vi "Get Joystick Values.vi"(8 "error in (no error)":errorcluster, 11 "One Driver in":refnum<class "One Driver.lvclass">) -> (0 "error out":errorcluster, 2 "Joystick Data":T1, 3 "One Driver out":refnum<class "One Driver.lvclass">)   [LabVIEW 2018, in "Joysticks.lvlib" / "One Driver.lvclass"]
doc: "Use this method to get the joystick values in a cluster you can use for your application.\n\nModify the Type Def that this VI resturns to fit the controls needed for the robot."
uses:
  One Driver.lvclass
  C:/Users/Public/Documents/2019DeepSpace/Classes/Joysticks/Joysticks.lvclass
  Controls/JoystickData.ctl
  One Driver.lvclass/One Driver.ctl
  Joysticks.lvclass/Joysticks.ctl
  Public Methods/Read Sensitivity(x).vi
  Public Methods/Read Sensitivity(y).vi
  <vilib>/Rock Robotics/WPI/Utilities/WPI_GetSetVariantRefNum.vi
  Private Methods/POV Conditioning.vi
  Joysticks.lvclass
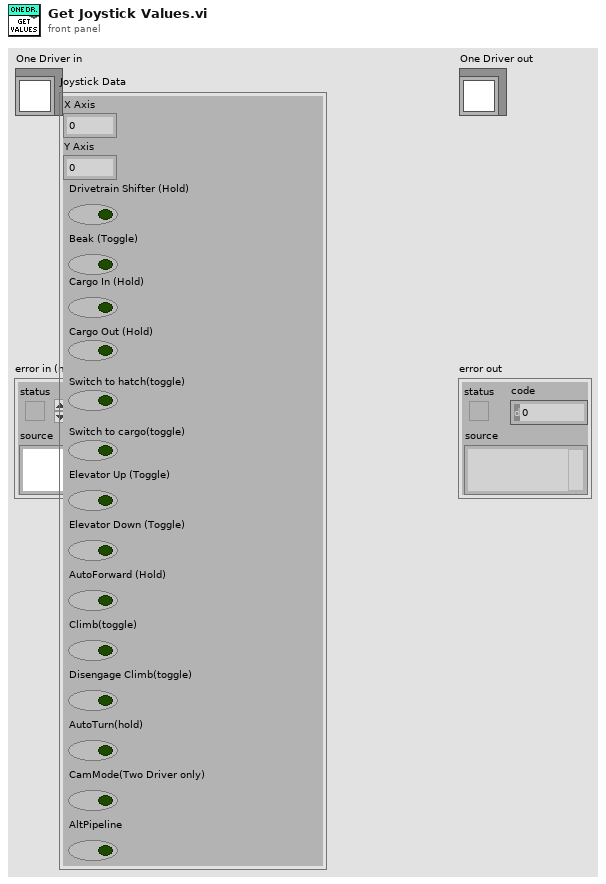
[diagram p1: front panel]
types:
  T1 = typedef "Joysticks.lvlib/Joysticks.lvclass/JoystickData.ctl" = cluster{"X Axis":dbl, "Y Axis":dbl, "Drivetrain Shifter (Hold)":bool, "Beak (Toggle)":bool, "Cargo In (Hold)":bool, "Cargo Out (Hold)":bool, "Switch to hatch(toggle)":bool, "Switch to cargo(toggle)":bool, "Elevator Up (Toggle)":bool, "Elevator Down (Toggle)":bool, "AutoForward (Hold)":bool, "Climb(toggle)":bool, "Disengage Climb(toggle)":bool, "AutoTurn(hold)":bool, "CamMode(Two Driver only)":bool, "AltPipeline":bool}
  T2 = typedef "WPI_JoystickDevRef.ctl" = cluster{"Device":T3}
  T3 = typedef "WPI_JoystickDeviceEnum.ctl" = enum16{"USB 0", "USB 1", "USB 2", "USB 3", "USB 4", "USB 5"}
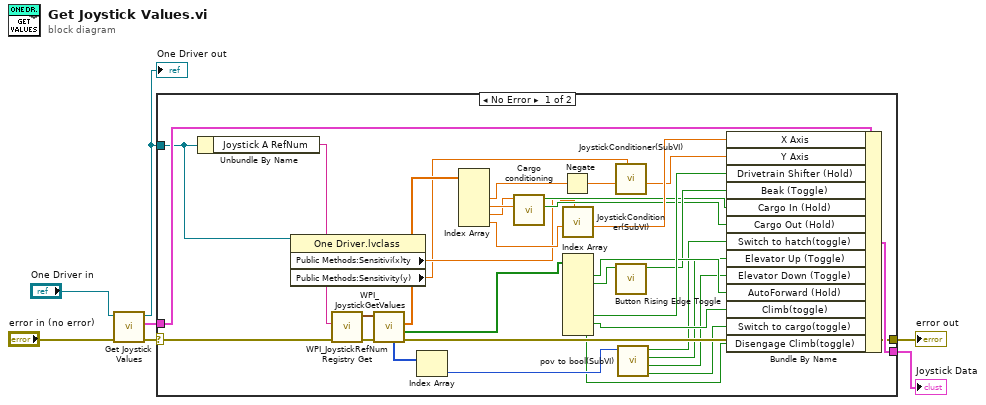
[diagram p0: block diagram]
diagram:
  n1 = call-parent "Get Joystick Values.vi"("error in (no error)"="error in (no error)", "Joysticks in"="One Driver in") -> ("error out"=w2:errorcluster, "Joystick Data"=w5:T1, "Joysticks out"=w1:refnum<class "One Driver.lvclass">)  [unwired: 7 in]
  "One Driver out" <- w1
  n2 = case shown="No Error" w2 {
    selector: w2 -> [w40 w41]
    tunnel: [w30 w41] -> w7
    tunnel: w1 -> [w11 _]
    tunnel: [w36 _] -> w6
    tunnel: w5 -> [w31 _]
    frame No Error {
      n3 = Unbundle By Name(w11) -> ("Joystick A RefNum"=w38:string)
      n4 = property class="One Driver.lvclass"(reference=w11) -> ("Public Methods:Sensitivi(x)ty"=w10:dbl, "Public Methods:Sensitivity(y)"=w9:dbl)  [unwired: 1 in, 2 out]
      n5 = call <vilib>:"WPI_JoystickRefNum Registry Get.vi"("error in (no error)"=w40, "refnum name"=w38) -> ("error out"=w39:errorcluster, "JoystickDevRef"=w37:T2)  [unwired: 8 in]
      n6 = call <vilib>:"WPI_JoystickGetValues.vi"("error in (no error)"=w39, "JoystickDevRef"=w37) -> ("error out"=w30:errorcluster, "Buttons"=w35:bool[], "Axes"=w34:dbl[], "POVs"=w25:i16[])  [unwired: 5 in, 1 out]
      n7 = Index Array(array=w25) -> (element=w16:i16)  [unwired: 1 in]
      n8 = Index Array(array=w34) -> (element #2=w32:dbl, element #3=w18:dbl, element #4=w17:dbl, element #5=w29:dbl)  [unwired: 5 in, 1 out]
      n9 = call "Cargo conditioning.vi"("Cargo Out (Axis)"=w18, "Cargo In (Axis)"=w17) -> ("Cargo Out (Hold)"=w20:bool, "Cargo In (Hold)"=w19:bool)  [unwired: 8 in]
      n10 = Negate(x=w32) -> (-x=w27:dbl)
      n11 = call "JoystickConditioner(SubVI).vi"("Sensitivity"=w10, "joystick axis"=w29) -> ("output"=w28:dbl)  [unwired: 9 in]
      n12 = Index Array(array=w35) -> (element #1=w24:bool, element #2=w22:bool, element #6=w33:bool, element #7=w21:bool, element #8=w8:bool)  [unwired: 8 in, 3 out]
      n13 = call "JoystickConditioner(SubVI).vi"("Sensitivity"=w9, "joystick axis"=w27) -> ("output"=w26:dbl)  [unwired: 9 in]
      n14 = call "Button Rising Edge Toggle.vi"("Button"=w22) -> ("Rising edge?"=w23:bool)  [unwired: 10 in]
      n15 = call "pov to bool(SubVI).vi"("Numeric"=w16) -> ("Left"=w12:bool, "Down"=w13:bool, "Up"=w14:bool, "Right"=w15:bool)  [unwired: 7 in]
      n16 = Bundle By Name(cluster=w31, "X Axis"=w28, "Y Axis"=w26, "Drivetrain Shifter (Hold)"=w33, "Beak (Toggle)"=w23, "Cargo In (Hold)"=w19, "Cargo Out (Hold)"=w20, "Switch to hatch(toggle)"=w15, "Elevator Up (Toggle)"=w14, "Elevator Down (Toggle)"=w13, "AutoForward (Hold)"=w24, "Climb(toggle)"=w21, "Switch to cargo(toggle)"=w12, "Disengage Climb(toggle)"=w8) -> (w36:T1)
    }
    frame Error {
    }
  }
  "error out" <- w7
  "Joystick Data" <- w6
